vi "Create.vi"   [LabVIEW 2018, in "Toolkit.lvlib" / "Agent Identity.lvclass"]
uses:
  Agent Identity.lvclass
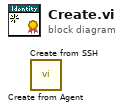
[diagram p0: block diagram]
diagram:
  n1 = call "Create from Agent.vi"() -> ()  [unwired: 9 in, 3 out]
  n2 = call "Create from SSH.vi"() -> ()  [unwired: 10 in, 2 out]
